vi "Write parent.vi"(8 "error in (no error)":errorcluster, 10 "parent":refnum<k24>, 11 "[MDI] Child in":refnum<class "[MDI] Child.lvclass">) -> (0 "error out":errorcluster, 3 "[MDI] Child out":refnum<class "[MDI] Child.lvclass">)   [LabVIEW 2020, in "[MDI] Child.lvlib" / "[MDI] Child.lvclass"]
uses:
  [MDI] Child.lvclass
  System.Windows.Forms
  [MDI] Child.lvclass/[MDI] Child.ctl
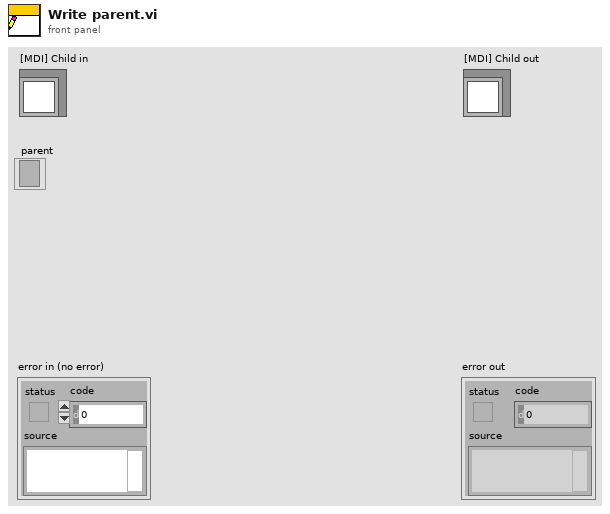
[diagram p1: front panel]
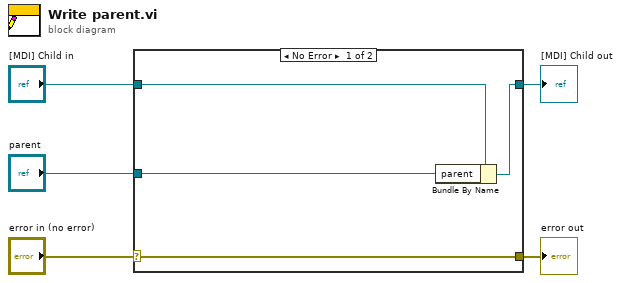
[diagram p0: block diagram]
diagram:
  n1 = case shown="No Error" "error in (no error)" {
    selector: "error in (no error)" -> [w9 w10]
    tunnel: [w9 w10] -> w4
    tunnel: [w7 w11] -> w2
    tunnel: "[MDI] Child in" -> [w8 w11]
    tunnel: "parent" -> [w6 _]
    frame No Error {
      n2 = Bundle By Name(cluster=w8, "parent"=w6) -> (w7:refnum<class "[MDI] Child.lvclass">)
    }
    frame Error {
    }
  }
  "error out" <- w4
  "[MDI] Child out" <- w2
